vi "test - Round Trip - Array - Boolean.vi"(8 "error in (no error)":errorcluster, 11 "TestCase in":refnum<class "Python Data Tools Tests.lvclass">) -> (0 "error out":errorcluster, 3 "TestCase out":refnum<class "Python Data Tools Tests.lvclass">)   [LabVIEW 2013, in "Python Data Tools Tests.lvclass"]
uses:
  Python Data Tools Tests.lvclass
  <vilib>/addons/_JKI Toolkits/VI Tester/TestCase.llb/TestCase.lvclass
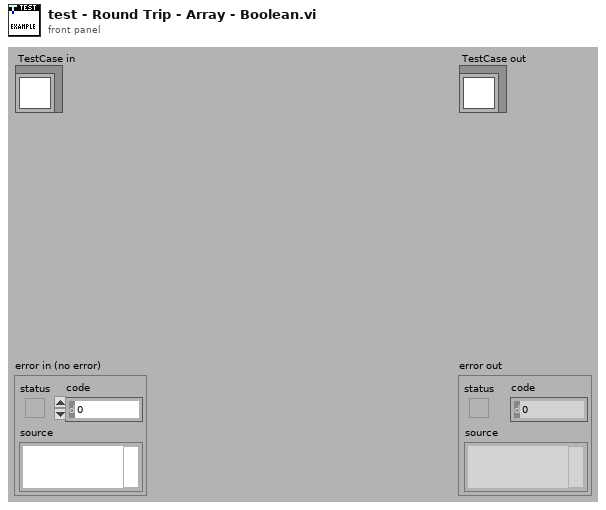
[diagram p1: front panel]
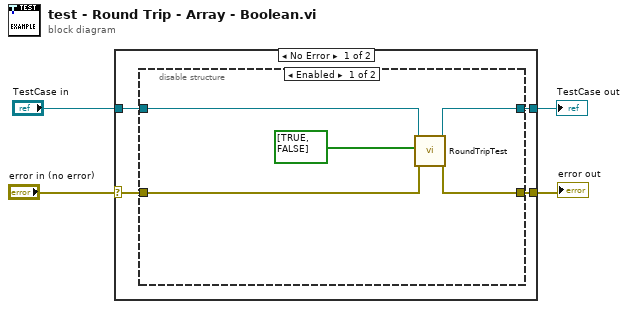
[diagram p0: block diagram]
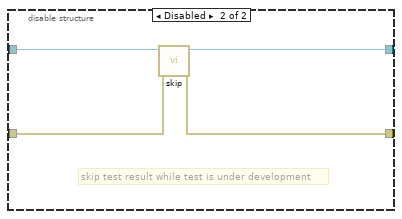
[diagram p2: hidden frame]
diagram:
  n1 = case shown="No Error" "error in (no error)" {
    selector: "error in (no error)" -> [w6 w19]
    tunnel: [w5 w19] -> w3
    tunnel: [w7 w18] -> w1
    tunnel: "TestCase in" -> [w8 w18]
    frame No Error {
      n2 = disable-structure shown="Enabled" {
        disable-tunnel: w8 -> [w13 w17]
        disable-tunnel: [w12 w14] -> w7
        disable-tunnel: w6 -> [w10 w16]
        disable-tunnel: [w11 w15] -> w5
        frame Enabled {
          n3 = call "RoundTripTest.vi"("error in (no error)"=w10, "Variant"=bool[] [TRUE, FALSE], "TestCase in"=w13) -> ("error out"=w11:errorcluster, "TestCase out"=w12:refnum<class "Python Data Tools Tests.lvclass">)  [unwired: 6 in, 1 out]
        }
        frame Disabled {
          # "skip test result while test is under development"
          n4 = call <vilib>:"skip.vi"("error in (no error)"=w16, "TestCase in"=w17) -> ("error out"=w15:errorcluster, "TestCase out"=w14:refnum<class "Python Data Tools Tests.lvclass">)  [unwired: 8 in]
        }
      }
    }
    frame Error {
    }
  }
  "error out" <- w3
  "TestCase out" <- w1
